vi "Init.vi"(8 "error in (no error)":errorcluster, 10 "VMR":refnum<class "VMR.lvclass">) -> (0 "error out":errorcluster, 3 "WebServer out":refnum<class "WebServer.lvclass">)   [LabVIEW 2022 SP3, in "VMR-Deck.lvlib" / "WebServer.lvclass"]
uses:
  WebServer.lvclass
  WebServer.lvclass/WebServer.ctl
  <vilib>/IlluminatedG/IG HTTP Server/HTTP Server/Server/Server.lvclass
  VMR/VMR.lvclass
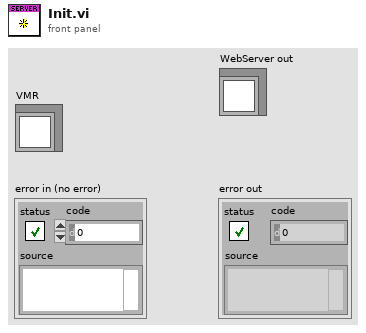
[diagram p1: front panel]
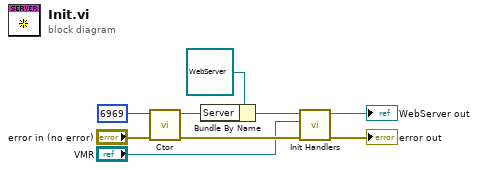
[diagram p0: block diagram]
diagram:
  n1 = call <vilib>:"Ctor.vi"("error in (no error)"="error in (no error)", "HTTP Port (80)"=u16 6969) -> ("error out"=w5:errorcluster, "Server out"=w6:refnum<class "Server.lvclass">)  [unwired: 8 in]
  n2 = Bundle By Name(cluster=refnum<class "WebServer.lvclass"> refnum ("WebServer in"), "Server"=w6) -> (w3:refnum<class "WebServer.lvclass">)
  n3 = call "Init Handlers.vi"("error in (no error)"=w5, "VMR"="VMR", "WebServer in"=w3) -> ("error out"=→"error out":errorcluster, "WebServer out"=→"WebServer out":refnum<class "WebServer.lvclass">)  [unwired: 7 in]
